vi "Store Value.vi"(7 "Numeric":i64, 8 "Memory in":cluster{"w":i64, "x":i64, "y":i64, "z":i64}, 11 "String":string) -> (0 "Memory out":cluster{"w":i64, "x":i64, "y":i64, "z":i64})   [LabVIEW 2021]
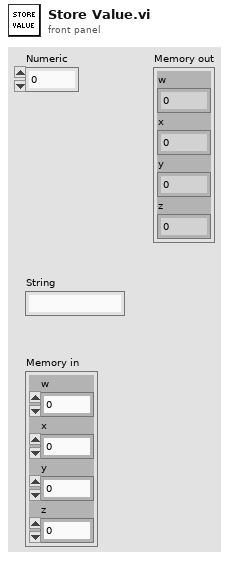
[diagram p1: front panel]
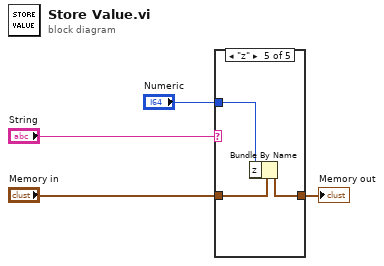
[diagram p0: block diagram]
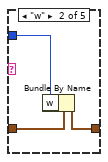
[diagram p3: hidden frame]
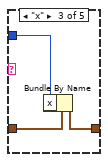
[diagram p4: hidden frame]
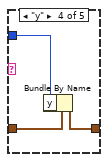
[diagram p5: hidden frame]
diagram:
  n1 = case shown="\"z\"" "String" {
    tunnel: "Memory in" -> [w5 w8 w11 w14 w17]
    tunnel: [w5 w7 w10 w13 w16] -> w3
    tunnel: "Numeric" -> [_ w6 w9 w12 w15]
    frame Default {
    }
    frame "w" {
      n2 = Bundle By Name(cluster=w8, "w"=w6) -> (w7:cluster{"w":i64, "x":i64, "y":i64, "z":i64})
    }
    frame "x" {
      n3 = Bundle By Name(cluster=w11, "x"=w9) -> (w10:cluster{"w":i64, "x":i64, "y":i64, "z":i64})
    }
    frame "y" {
      n4 = Bundle By Name(cluster=w14, "y"=w12) -> (w13:cluster{"w":i64, "x":i64, "y":i64, "z":i64})
    }
    frame "z" {
      n5 = Bundle By Name(cluster=w17, "z"=w15) -> (w16:cluster{"w":i64, "x":i64, "y":i64, "z":i64})
    }
  }
  "Memory out" <- w3
